vi "Dequeue Message.vi"(8 "error in (no error)":errorcluster, 11 "Message Queue":refnum<queue>) -> (0 "error out":errorcluster, 1 "output data":dbl[][](array[numeric]), 2 "Message":string, 3 "dup Message Queue":refnum<queue>)   [LabVIEW 2025, in "LAB-IQ Message Queue.lvlib"]
doc: "This VI pulls messages off the Message Queue."
uses:
  LAB-IQ Message Queue.lvlib
  Message Cluster.ctl
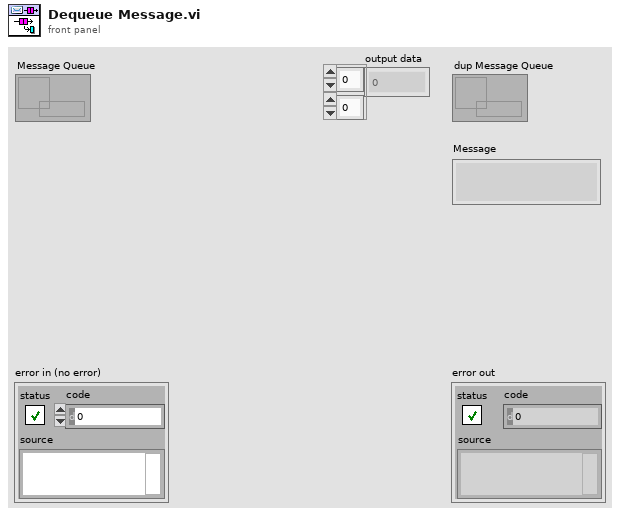
[diagram p1: front panel]
types:
  T1 = typedef "LAB-IQ Message Queue.lvlib/Message Cluster.ctl" = cluster{"Message":string, "output data":dbl[][]}
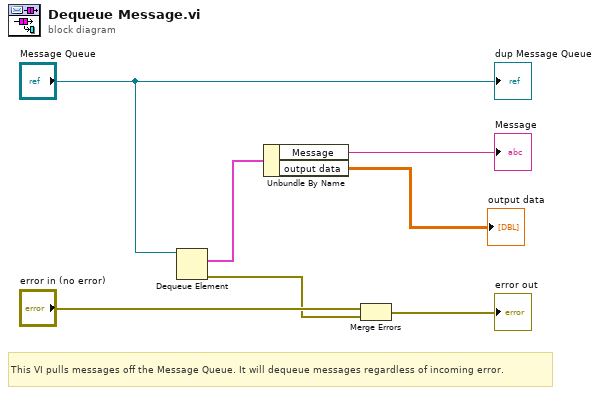
[diagram p0: block diagram]
diagram:
  # "This VI pulls messages off the Message Queue. It will dequeue messages regardless of incoming error."
  n1 = Dequeue Element(queue="Message Queue") -> (element=w5:T1, error out=w2:errorcluster)  [unwired: 2 in, 2 out]
  n2 = Unbundle By Name(w5) -> ("Message"=→"Message":string, "output data"=→"output data":dbl[][])
  n3 = Merge Errors("error in (no error)", w2) -> (→"error out":errorcluster)
  "dup Message Queue" <- "Message Queue"
